vi "Write_LS_Data.vi"(1 "In":T1={"Time"=[], "LI1CH1"=[], "LI1CH2"=[], "LI2CH1"=[], "LI2CH2"=[], "LI3CH1"=[], "LI3CH2"=[], "Field"=[], "Temperature"=[], "Temperature 2"=[], "Temperatrue 3"=[], "Nitrogen_Level"=[], "Helium_Level"=[], "Heater_LS370"=[], "Sorb_Heater"=[], "Still_Heater"=[], "Capacity"=[], "Loss"=[], "Magnet_Temperature"=[], "Lambda_Pressure"=[], "Lambda_Needle_Valve"=[], "LS370-CH1-T"=[], "LS370-CH2-T"=[], "LS370-CH3-T"=[], "LS370-CH4-T"=[], "LS370-TC-T"=[], "LS370-CH1-R"=[], "LS370-CH2-R"=[], "LS370-CH3-R"=[], "LS370-CH4-R"=[], "LS370-TC-R"=[], "LS372-CH1-T"=[], "LS372-CH2-T"=[], "LS372-CH3-T"=[], "LS372-CH4-T"=[], "LS372-CH5-T"=[], "LS372-CH1-R"=[], "LS372-CH2-R"=[], "LS372-CH3-R"=[], "LS372-CH4-R"=[], "LS372-CH5-R"=[], "Nada"=[nan], "Keithley_Res"=[], "Keithley_Current"=[], "VTI_Heater"=[], "VTI_Needle Valve"=[], "LS340_Heater"=[], "Keithley_6221_Amplitude"=[], "Keithley_6221_Frequency"=[], "Condense_Pressure"=[], "Still_Pressure"=[], "FP_Out_Pressure"=[], "Dump_Pressure"=[], "V1"=[], "V2"=[], "V4"=[], "V5"=[], "V9"=[], "Forepump"=[], "Compressor"=[], "Keihtley_6221_Offset"=[], "BoxTemp"=[], "By"=[], "Bz"=[], "Phi"=[], "heater-recond (%)"=[], "Dewar Pressure "=[]}) -> (0 "Out":T1={"Time"=[], "LI1CH1"=[], "LI1CH2"=[], "LI2CH1"=[], "LI2CH2"=[], "LI3CH1"=[], "LI3CH2"=[], "Field"=[], "Temperature"=[], "Temperature 2"=[], "Temperatrue 3"=[], "Nitrogen_Level"=[], "Helium_Level"=[], "Heater_LS370"=[], "Sorb_Heater"=[], "Still_Heater"=[], "Capacity"=[], "Loss"=[], "Magnet_Temperature"=[], "Lambda_Pressure"=[], "Lambda_Needle_Valve"=[], "LS370-CH1-T"=[], "LS370-CH2-T"=[], "LS370-CH3-T"=[], "LS370-CH4-T"=[], "LS370-TC-T"=[], "LS370-CH1-R"=[], "LS370-CH2-R"=[], "LS370-CH3-R"=[], "LS370-CH4-R"=[], "LS370-TC-R"=[], "LS372-CH1-T"=[], "LS372-CH2-T"=[], "LS372-CH3-T"=[], "LS372-CH4-T"=[], "LS372-CH5-T"=[], "LS372-CH1-R"=[], "LS372-CH2-R"=[], "LS372-CH3-R"=[], "LS372-CH4-R"=[], "LS372-CH5-R"=[], "Nada"=[nan], "Keithley_Res"=[], "Keithley_Current"=[], "VTI_Heater"=[], "VTI_Needle Valve"=[], "LS340_Heater"=[], "Keithley_6221_Amplitude"=[], "Keithley_6221_Frequency"=[], "Condense_Pressure"=[], "Still_Pressure"=[], "FP_Out_Pressure"=[], "Dump_Pressure"=[], "V1"=[], "V2"=[], "V4"=[], "V5"=[], "V9"=[], "Forepump"=[], "Compressor"=[], "Keihtley_6221_Offset"=[], "BoxTemp"=[], "By"=[], "Bz"=[], "Phi"=[], "heater-recond (%)"=[], "Dewar Pressure "=[]})   [LabVIEW 2016]
uses:
  Global/Global Variables/System Monitor Cluster.ctl
  Global/Global Variables/Data_Display_global.vi
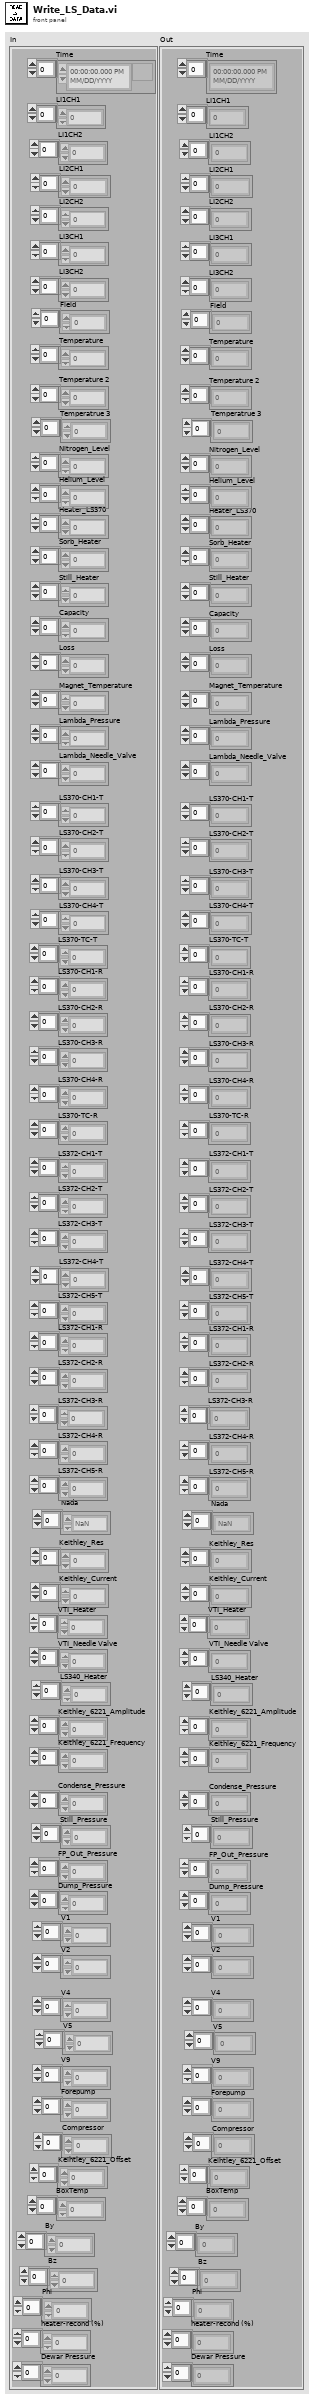
[diagram p1: front panel]
types:
  T1 = typedef "System Monitor Cluster.ctl" = cluster{"Time":timestamp[], "LI1CH1":dbl[], "LI1CH2":dbl[], "LI2CH1":dbl[], "LI2CH2":dbl[], "LI3CH1":dbl[], "LI3CH2":dbl[], "Field":dbl[], "Temperature":dbl[], "Temperature 2":dbl[], "Temperatrue 3":dbl[], "Nitrogen_Level":dbl[], "Helium_Level":dbl[], "Heater_LS370":dbl[], "Sorb_Heater":dbl[], "Still_Heater":dbl[], "Capacity":dbl[], "Loss":dbl[], "Magnet_Temperature":dbl[], "Lambda_Pressure":dbl[], "Lambda_Needle_Valve":dbl[], "LS370-CH1-T":dbl[], "LS370-CH2-T":dbl[], "LS370-CH3-T":dbl[], "LS370-CH4-T":dbl[], "LS370-TC-T":dbl[], "LS370-CH1-R":dbl[], "LS370-CH2-R":dbl[], "LS370-CH3-R":dbl[], "LS370-CH4-R":dbl[], "LS370-TC-R":dbl[], "LS372-CH1-T":dbl[], "LS372-CH2-T":dbl[], "LS372-CH3-T":dbl[], "LS372-CH4-T":dbl[], "LS372-CH5-T":dbl[], "LS372-CH1-R":dbl[], "LS372-CH2-R":dbl[], "LS372-CH3-R":dbl[], "LS372-CH4-R":dbl[], "LS372-CH5-R":dbl[], "Nada":dbl[], "Keithley_Res":dbl[], "Keithley_Current":dbl[], "VTI_Heater":dbl[], "VTI_Needle Valve":dbl[], "LS340_Heater":dbl[], "Keithley_6221_Amplitude":dbl[], "Keithley_6221_Frequency":dbl[], "Condense_Pressure":dbl[], "Still_Pressure":dbl[], "FP_Out_Pressure":dbl[], "Dump_Pressure":dbl[], "V1":dbl[], "V2":dbl[], "V4":dbl[], "V5":dbl[], "V9":dbl[], "Forepump":dbl[], "Compressor":dbl[], "Keihtley_6221_Offset":dbl[], "BoxTemp":dbl[], "By":dbl[], "Bz":dbl[], "Phi":dbl[], "heater-recond (%)":dbl[], "Dewar Pressure ":dbl[]}
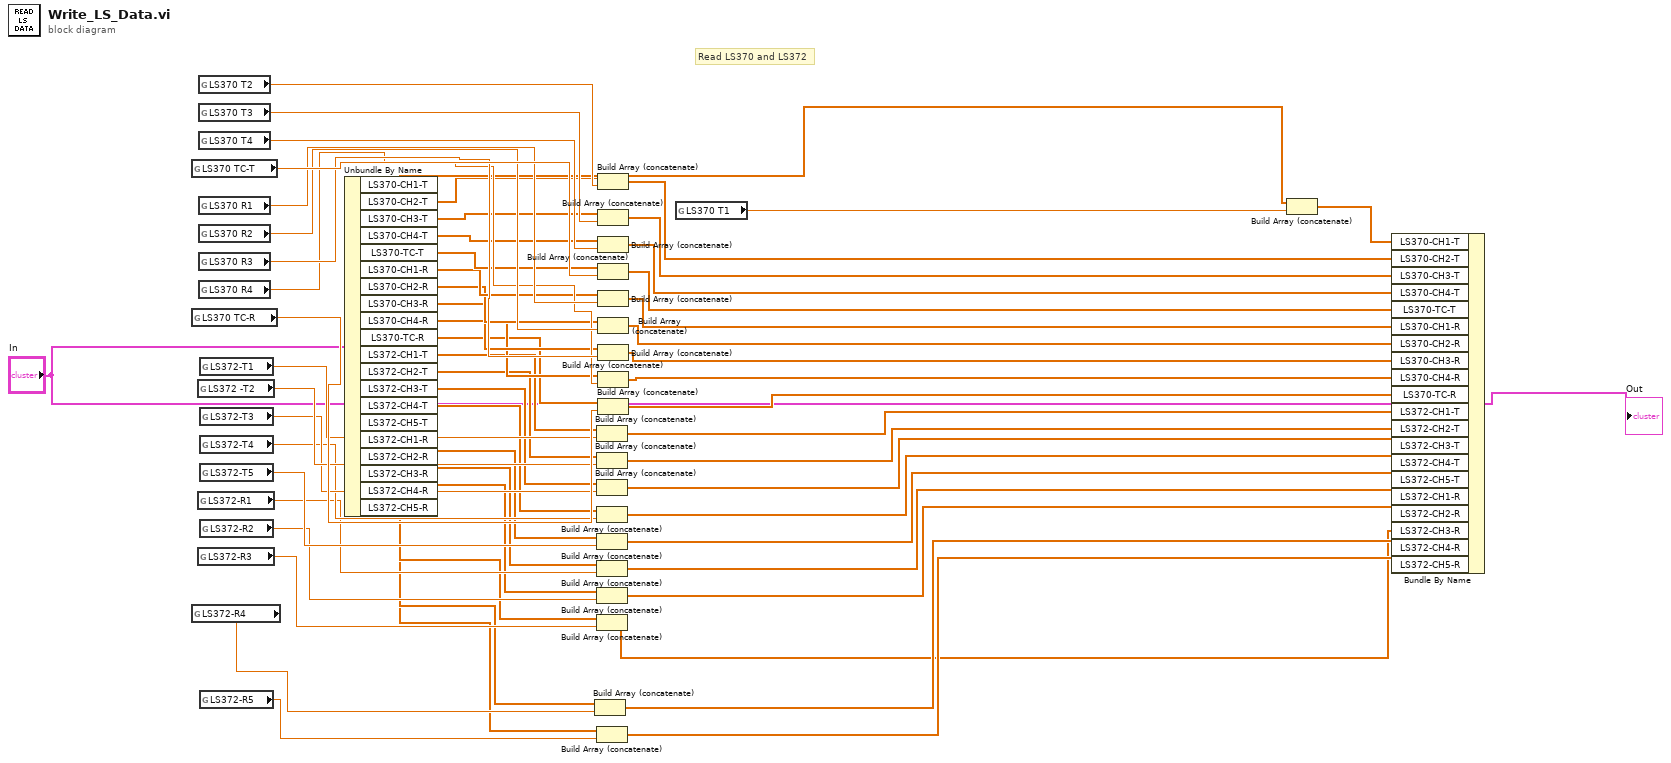
[diagram p0: block diagram]
diagram:
  # "Read LS370 and LS372"
  n1 = global read "Data_Display_global.vi" "LS370 TC-T"() -> (w58:dbl)
  n2 = global read "Data_Display_global.vi" "LS370 TC-R"() -> (w53:dbl)
  n3 = global read "Data_Display_global.vi" "LS372-R4"() -> (w44:dbl)
  n4 = global read "Data_Display_global.vi" "LS372 -T2"() -> (w51:dbl)
  n5 = global read "Data_Display_global.vi" "LS372-R1"() -> (w47:dbl)
  n6 = global read "Data_Display_global.vi" "LS372-R3"() -> (w45:dbl)
  n7 = global read "Data_Display_global.vi" "LS370 T2"() -> (w61:dbl)
  n8 = global read "Data_Display_global.vi" "LS370 T3"() -> (w60:dbl)
  n9 = global read "Data_Display_global.vi" "LS370 T4"() -> (w59:dbl)
  n10 = global read "Data_Display_global.vi" "LS370 R1"() -> (w57:dbl)
  n11 = global read "Data_Display_global.vi" "LS370 R2"() -> (w56:dbl)
  n12 = global read "Data_Display_global.vi" "LS370 R3"() -> (w55:dbl)
  n13 = global read "Data_Display_global.vi" "LS370 R4"() -> (w54:dbl)
  n14 = global read "Data_Display_global.vi" "LS372-T1"() -> (w52:dbl)
  n15 = global read "Data_Display_global.vi" "LS372-T3"() -> (w50:dbl)
  n16 = global read "Data_Display_global.vi" "LS372-T4"() -> (w49:dbl)
  n17 = global read "Data_Display_global.vi" "LS372-T5"() -> (w48:dbl)
  n18 = global read "Data_Display_global.vi" "LS372-R2"() -> (w46:dbl)
  n19 = global read "Data_Display_global.vi" "LS372-R5"() -> (w43:dbl)
  n20 = Unbundle By Name("In") -> ("LS370-CH1-T"=w42:dbl[], "LS370-CH2-T"=w41:dbl[], "LS370-CH3-T"=w40:dbl[], "LS370-CH4-T"=w39:dbl[], "LS370-TC-T"=w38:dbl[], "LS370-CH1-R"=w37:dbl[], "LS370-CH2-R"=w36:dbl[], "LS370-CH3-R"=w35:dbl[], "LS370-CH4-R"=w34:dbl[], "LS370-TC-R"=w33:dbl[], "LS372-CH1-T"=w32:dbl[], "LS372-CH2-T"=w31:dbl[], "LS372-CH3-T"=w30:dbl[], "LS372-CH4-T"=w29:dbl[], "LS372-CH5-T"=w28:dbl[], "LS372-CH1-R"=w27:dbl[], "LS372-CH2-R"=w26:dbl[], "LS372-CH3-R"=w25:dbl[], "LS372-CH4-R"=w24:dbl[], "LS372-CH5-R"=w23:dbl[])
  n21 = Build Array (concatenate)(w24, w44) -> (w5:dbl[])
  n22 = Build Array (concatenate)(w32, w52) -> (w12:dbl[])
  n23 = Build Array (concatenate)(w31, w51) -> (w11:dbl[])
  n24 = Build Array (concatenate)(w30, w50) -> (w10:dbl[])
  n25 = Build Array (concatenate)(w29, w49) -> (w9:dbl[])
  n26 = Build Array (concatenate)(w28, w48) -> (w8:dbl[])
  n27 = Build Array (concatenate)(w27, w47) -> (w7:dbl[])
  n28 = Build Array (concatenate)(w26, w46) -> (w6:dbl[])
  n29 = Build Array (concatenate)(w25, w45) -> (w1:dbl[])
  n30 = Build Array (concatenate)(w23, w43) -> (w4:dbl[])
  n31 = Build Array (concatenate)(w41, w61) -> (w21:dbl[])
  n32 = Build Array (concatenate)(w40, w60) -> (w20:dbl[])
  n33 = Build Array (concatenate)(w39, w59) -> (w19:dbl[])
  n34 = Build Array (concatenate)(w38, w58) -> (w18:dbl[])
  n35 = Build Array (concatenate)(w37, w57) -> (w17:dbl[])
  n36 = Build Array (concatenate)(w36, w56) -> (w16:dbl[])
  n37 = Build Array (concatenate)(w35, w55) -> (w15:dbl[])
  n38 = Build Array (concatenate)(w34, w54) -> (w14:dbl[])
  n39 = Build Array (concatenate)(w33, w53) -> (w13:dbl[])
  n40 = global read "Data_Display_global.vi" "LS370 T1"() -> (w62:dbl)
  n41 = Build Array (concatenate)(w42, w62) -> (w22:dbl[])
  n42 = Bundle By Name(cluster="In", "LS370-CH1-T"=w22, "LS370-CH2-T"=w21, "LS370-CH3-T"=w20, "LS370-CH4-T"=w19, "LS370-TC-T"=w18, "LS370-CH1-R"=w17, "LS370-CH2-R"=w16, "LS370-CH3-R"=w15, "LS370-CH4-R"=w14, "LS370-TC-R"=w13, "LS372-CH1-T"=w12, "LS372-CH2-T"=w11, "LS372-CH3-T"=w10, "LS372-CH4-T"=w9, "LS372-CH5-T"=w8, "LS372-CH1-R"=w7, "LS372-CH2-R"=w6, "LS372-CH3-R"=w1, "LS372-CH4-R"=w5, "LS372-CH5-R"=w4) -> (→"Out":T1)
